vi "PLAN IN FEEDING SCREEN.vi"(10 "Section selected":i32, 11 "PLAN In":string[][](array[string])) -> (0 "FEED CMPLT?":bool, 1 "Bin/Box":i32, 2 "PLAN Out":string[][](array[string]), 3 "CURRENT PLAN":T1)   [LabVIEW 2017]
panel:
  # "DOOR NUMBER"
  # "FEEDER STATUS"
  # "DOOR NUMBER"
  # "FEEDER STATUS"
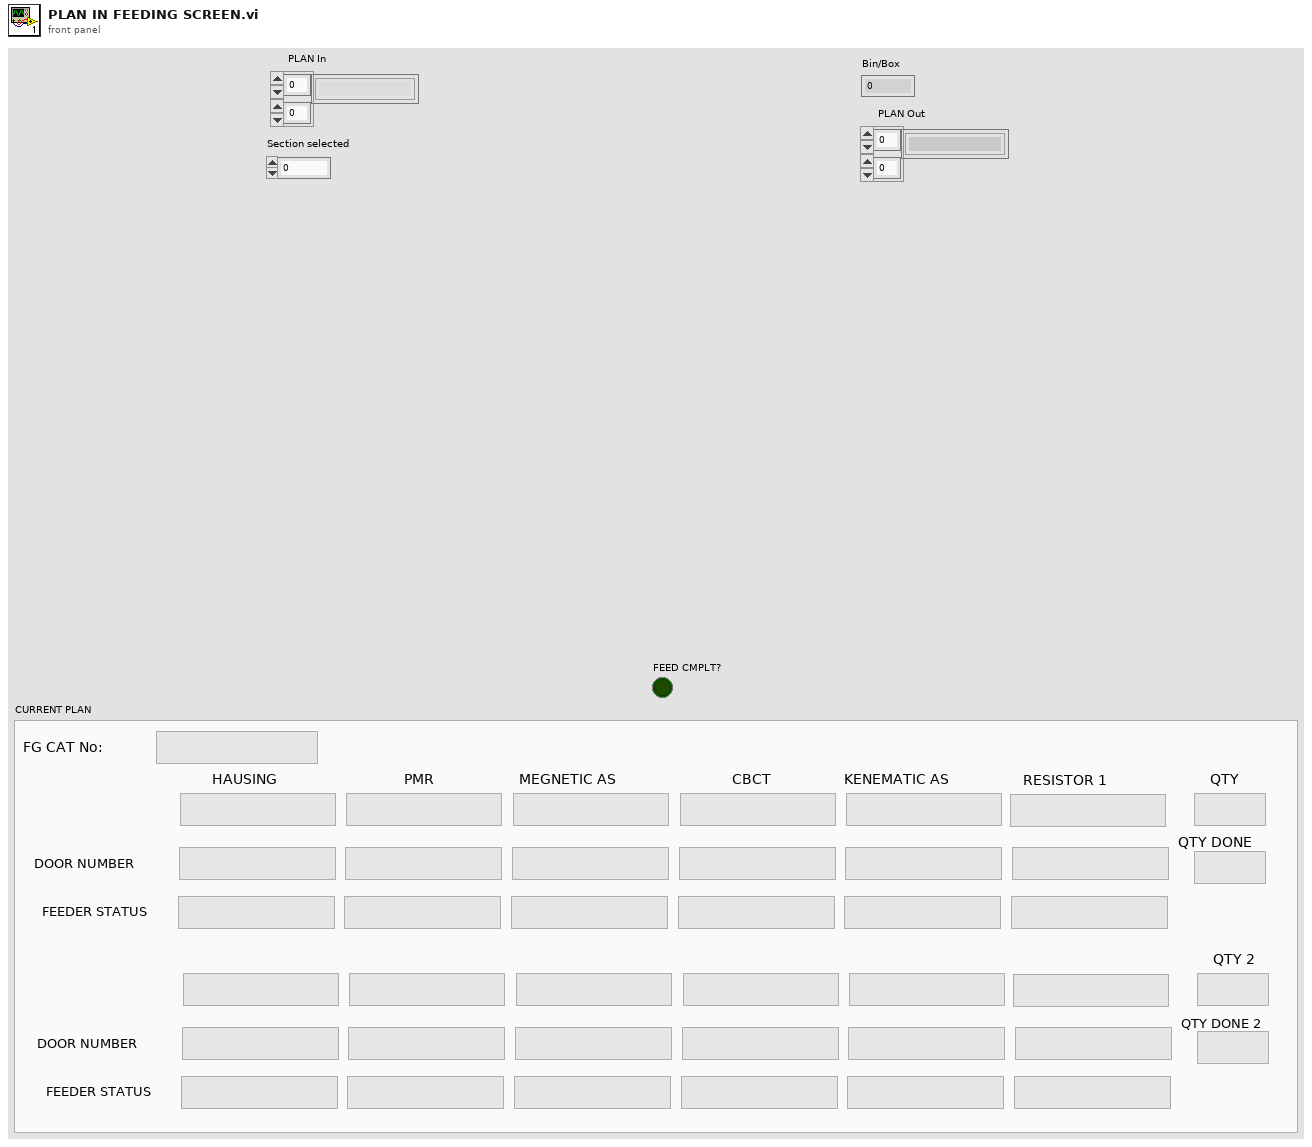
[diagram p1: front panel]
types:
  T1 = cluster{"FG CAT No:":string, "HAUSING":string, "PMR":string, "MEGNETIC AS":string, "CBCT":string, "KENEMATIC AS":string, "RESISTOR 1":string, "HAUSING DOOR":string, "PMR DOOR":string, "MAGNETIC AS DOOR":string, "CBCT DOOR":string, "KINEMATIC AS DOOR":string, "RESISTOR 1 DOOR":string, "HAUSING FEED STATUS":string, "PMR FEED STATUS":string, "MAGNETIC AS FEEED STATUS":string, "CBCT FEED STATUS":string, "KINEMATIC AS FEED STATUS":string, "RESISTOR 1 FEED STATUS":string, "QTY":string, "QTY DONE":string, "HAUSING 2":string, "PMR 2":string, "MEGNETIC AS 2":string, "CBCT 2":string, "KENEMATIC AS 2":string, "RESISTOR 2":string, "HAUSING DOOR 2":string, "PMR DOOR 2":string, "MAGNETIC AS DOOR 2":string, "CBCT DOOR 2":string, "KINEMATIC AS DOOR 2":string, "RESISTOR 1 DOOR 2":string, "HAUSING FEED STATUS 2":string, "PMR FEED STATUS 2":string, "MAGNETIC AS FEEED STATUS 2":string, "CBCT FEED STATUS 2":string, "KINEMATIC AS FEED STATUS 2":string, "RESISTOR 1 FEED STATUS 2":string, "QTY 2":string, "QTY DONE 2":string}
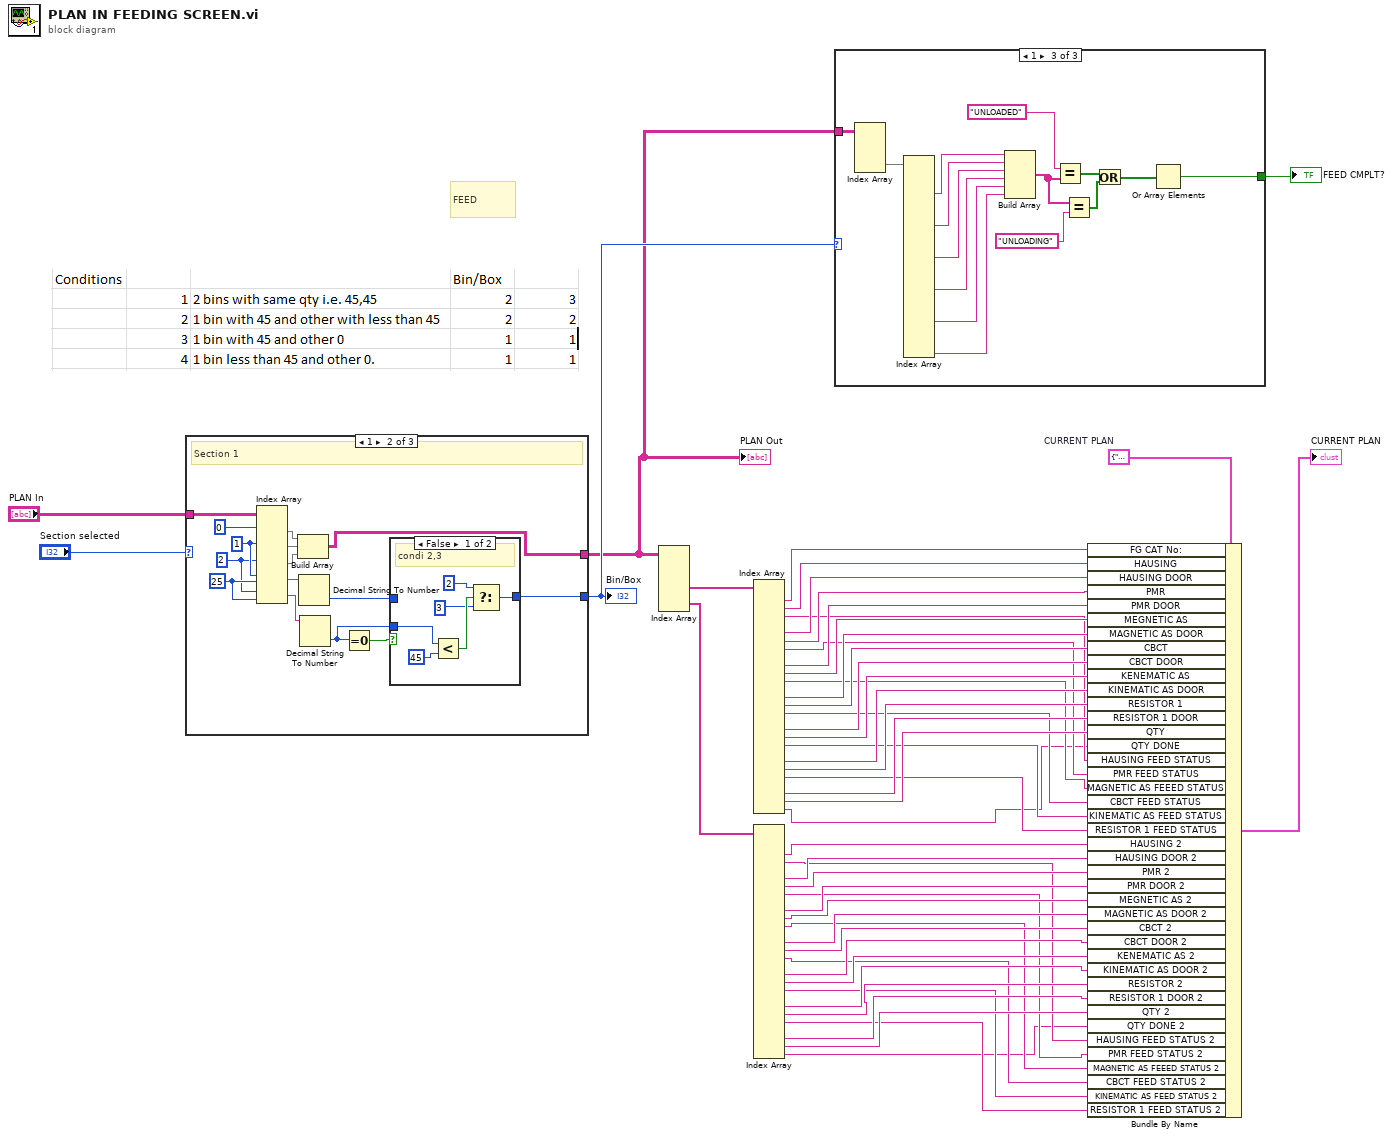
[diagram p0: block diagram]
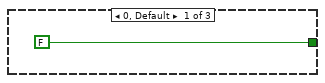
[diagram p2: hidden frame]
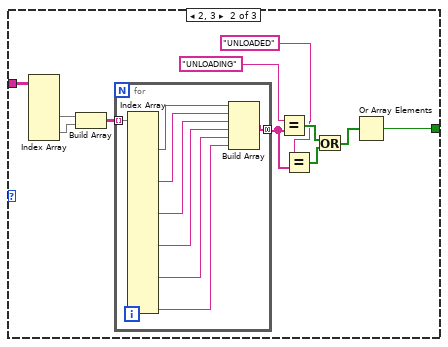
[diagram p3: hidden frame]
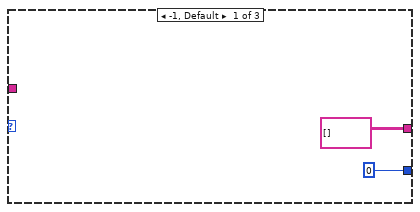
[diagram p4: hidden frame]
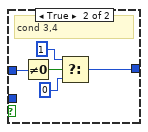
[diagram p5: hidden frame]
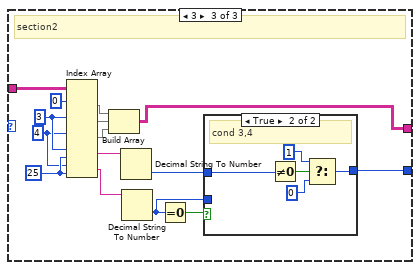
[diagram p6: hidden frame]
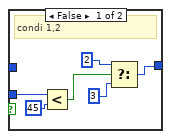
[diagram p7: hidden frame]
diagram:
  w4 = T1 {"FG CAT No:"="", "HAUSING"="", "PMR"="", "MEGNETIC AS"="", "CBCT"="", "KENEMATIC AS"="", "RESISTOR 1"="", "HAUSING DOOR"="", "PMR DOOR"="", "MAGNETIC AS DOOR"="", "CBCT DOOR"="", "KINEMATIC AS DOOR"="", "RESISTOR 1 DOOR"="", "HAUSING FEED STATUS"="", "PMR FEED STATUS"="", "MAGNETIC AS FEEED STATUS"="", "CBCT FEED STATUS"="", "KINEMATIC AS FEED STATUS"="", "RESISTOR 1 FEED STATUS"="", "QTY"="", "QTY DONE"="", "HAUSING 2"="", "PMR 2"="", "MEGNETIC AS 2"="", "CBCT 2"="", "KENEMATIC AS 2"="", "RESISTOR 2"="", "HAUSING DOOR 2"="", "PMR DOOR 2"="", "MAGNETIC AS DOOR 2"="", "CBCT DOOR 2"="", "KINEMATIC AS DOOR 2"="", "RESISTOR 1 DOOR 2"="", "HAUSING FEED STATUS 2"="", "PMR FEED STATUS 2"="", "MAGNETIC AS FEEED STATUS 2"="", "CBCT FEED STATUS 2"="", "KINEMATIC AS FEED STATUS 2"="", "RESISTOR 1 FEED STATUS 2"="", "QTY 2"="", "QTY DONE 2"=""}  # CURRENT PLAN
  # "FEED"
  n1 = case shown="1" "Section selected" {
    tunnel: "PLAN In" -> [_ w62 w93]
    tunnel: [string[][] [] w63 w89] -> w2
    tunnel: [0 w54 w87] -> w3
    frame -1, Default {
    }
    frame 1 {
      w60 = 25
      w59 = 2
      w61 = 1
      # "Section 1"
      n2 = Index Array(array=w62, index (row) #1=0, index (row) #2=w61, index (row) #3=w59, index (row) #4=w61, index (col) #4=w60, index (row) #5=w59, index (col) #5=w60) -> (element #1=w65:string[], element #2=w66:string[], element #3=w67:string[], element #4=w57:string, element #5=w58:string)  [unwired: 3 in]
      n3 = Build Array(w65, w66, w67) -> (w63:string[][])
      n4 = Decimal String To Number(string=w57) -> (number=w55:i32)  [unwired: 2 in, 1 out]
      n5 = Decimal String To Number(string=w58) -> (number=w53:i32)  [unwired: 2 in, 1 out]
      n6 = Equal To 0?(x=w53) -> (x = 0?=w56:bool)
      n7 = case shown="False" w56 {
        tunnel: w55 -> [_ w78]
        tunnel: [w71 w74] -> w54
        tunnel: w53 -> [w72 _]
        frame False {
          # "condi 2,3"
          n8 = Less?(x=w72, y=45) -> (x < y?=w69:bool)
          n9 = Select(t=2, s=w69, f=3) -> (s? t:f=w71:i32)
        }
        frame True {
          # "cond 3,4"
          n10 = Not Equal To 0?(x=w78) -> (x != 0?=w77:bool)
          n11 = Select(t=1, s=w77, f=0) -> (s? t:f=w74:i32)
        }
      }
    }
    frame 3 {
      w82 = 25
      w80 = 4
      w81 = 3
      # "section2"
      n12 = Index Array(array=w93, index (row) #1=0, index (row) #2=w81, index (row) #3=w80, index (row) #4=w81, index (col) #4=w82, index (row) #5=w80, index (col) #5=w82) -> (element #1=w92:string[], element #2=w91:string[], element #3=w90:string[], element #4=w84:string, element #5=w83:string)  [unwired: 3 in]
      n13 = Build Array(w92, w91, w90) -> (w89:string[][])
      n14 = Decimal String To Number(string=w84) -> (number=w86:i32)  [unwired: 2 in, 1 out]
      n15 = Decimal String To Number(string=w83) -> (number=w79:i32)  [unwired: 2 in, 1 out]
      n16 = Equal To 0?(x=w79) -> (x = 0?=w85:bool)
      n17 = case shown="True" w85 {
        tunnel: w86 -> [_ w104]
        tunnel: [w95 w100] -> w87
        tunnel: w79 -> [w94 _]
        frame False {
          # "condi 1,2"
          n18 = Less?(x=w94, y=45) -> (x < y?=w99:bool)
          n19 = Select(t=2, s=w99, f=3) -> (s? t:f=w95:i32)
        }
        frame True {
          # "cond 3,4"
          n20 = Not Equal To 0?(x=w104) -> (x != 0?=w103:bool)
          n21 = Select(t=1, s=w103, f=0) -> (s? t:f=w100:i32)
        }
      }
    }
  }
  "PLAN Out" <- w2
  "Bin/Box" <- w3
  n22 = Index Array(array=w2) -> (element #2=w50:string[], element #3=w35:string[])  [unwired: 6 in, 1 out]
  n23 = Index Array(array=w50) -> (element #1=w49:string, element #2=w48:string, element #3=w34:string, element #5=w47:string, element #6=w46:string, element #7=w33:string, element #9=w45:string, element #10=w44:string, element #11=w32:string, element #13=w43:string, element #14=w42:string, element #15=w31:string, element #17=w41:string, element #18=w40:string, element #19=w30:string, element #21=w39:string, element #22=w38:string, element #23=w29:string, element #25=w37:string, element #26=w36:string, element #27=w8:string)  [unwired: 27 in, 6 out]
  n24 = Index Array(array=w35) -> (element #2=w28:string, element #3=w15:string, element #5=w27:string, element #6=w26:string, element #7=w14:string, element #9=w25:string, element #10=w24:string, element #11=w13:string, element #13=w23:string, element #14=w22:string, element #15=w12:string, element #17=w21:string, element #18=w20:string, element #19=w11:string, element #21=w19:string, element #22=w18:string, element #23=w10:string, element #25=w17:string, element #26=w16:string, element #27=w7:string)  [unwired: 27 in, 7 out]
  n25 = case shown="1" w3 {
    tunnel: w2 -> [_ w116 w139]
    tunnel: [FALSE w111 w130] -> w1
    frame 0, Default {
    }
    frame 2, 3 {
      n26 = Index Array(array=w116) -> (element #2=w115:string[], element #3=w114:string[])  [unwired: 6 in, 1 out]
      n27 = Build Array(w115, w114) -> (w113:string[][])
      n28 = for {
        tunnel: w113 -> [w124] mode=indexing
        tunnel: [w117] -> w107 mode=concatenating
        n29 = Index Array(array=w124) -> (element #3=w123:string, element #7=w122:string, element #11=w121:string, element #15=w120:string, element #19=w119:string, element #23=w118:string)  [unwired: 23 in, 17 out]
        n30 = Build Array(w123, w122, w121, w120, w119, w118) -> (w117:string[])
      }
      n31 = Equal?(x="UNLOADING", y=w107) -> (x = y?=w109:bool[])
      n32 = Equal?(x="UNLOADED", y=w107) -> (x = y?=w110:bool[])
      n33 = Or(x=w109, y=w110) -> (x .or. y?=w108:bool[])
      n34 = Or Array Elements(Boolean array=w108) -> (logical OR=w111:bool)
    }
    frame 1 {
      n35 = Index Array(array=w139) -> (element #2=w138:string[])  [unwired: 4 in, 1 out]
      n36 = Index Array(array=w138) -> (element #3=w136:string, element #7=w135:string, element #11=w134:string, element #15=w133:string, element #19=w132:string, element #23=w131:string)  [unwired: 23 in, 17 out]
      n37 = Build Array(w136, w135, w134, w133, w132, w131) -> (w126:string[])
      n38 = Equal?(x="UNLOADED", y=w126) -> (x = y?=w129:bool[])
      n39 = Equal?(x=w126, y="UNLOADING") -> (x = y?=w125:bool[])
      n40 = Or(x=w129, y=w125) -> (x .or. y?=w128:bool[])
      n41 = Or Array Elements(Boolean array=w128) -> (logical OR=w130:bool)
    }
  }
  "FEED CMPLT?" <- w1
  n42 = Bundle By Name(cluster=w4, "FG CAT No:"=w49, "HAUSING"=w48, "HAUSING DOOR"=w47, "PMR"=w46, "PMR DOOR"=w45, "MEGNETIC AS"=w44, "MAGNETIC AS DOOR"=w43, "CBCT"=w42, "CBCT DOOR"=w41, "KENEMATIC AS"=w40, "KINEMATIC AS DOOR"=w39, "RESISTOR 1"=w38, "RESISTOR 1 DOOR"=w37, "QTY"=w36, "QTY DONE"=w8, "HAUSING FEED STATUS"=w34, "PMR FEED STATUS"=w33, "MAGNETIC AS FEEED STATUS"=w32, "CBCT FEED STATUS"=w31, "KINEMATIC AS FEED STATUS"=w30, "RESISTOR 1 FEED STATUS"=w29, "HAUSING 2"=w28, "HAUSING DOOR 2"=w27, "PMR 2"=w26, "PMR DOOR 2"=w25, "MEGNETIC AS 2"=w24, "MAGNETIC AS DOOR 2"=w23, "CBCT 2"=w22, "CBCT DOOR 2"=w21, "KENEMATIC AS 2"=w20, "KINEMATIC AS DOOR 2"=w19, "RESISTOR 2"=w18, "RESISTOR 1 DOOR 2"=w17, "QTY 2"=w16, "QTY DONE 2"=w7, "HAUSING FEED STATUS 2"=w15, "PMR FEED STATUS 2"=w14, "MAGNETIC AS FEEED STATUS 2"=w13, "CBCT FEED STATUS 2"=w12, "KINEMATIC AS FEED STATUS 2"=w11, "RESISTOR 1 FEED STATUS 2"=w10) -> (→"CURRENT PLAN":T1)
